vi "CODMn通讯.vi"() -> ()   [LabVIEW 2016, in "斯坦道CODMn.lvlib"]
uses:
  <vilib>/NI/Modbus Library/API/Wrapper/Create TCP Slave.vi
  <vilib>/NI/Modbus Library/API/slave/Modbus Slave.lvclass
  <vilib>/Plasmionique/MB Master/MB_Master/MB_Master.lvclass
  <vilib>/Plasmionique/MB Master/MB Master.lvlib
  <vilib>/Utility/config.llb/NI_LVConfig.lvlib
  <vilib>/NI/Modbus Library/API/Wrapper/API Main.lvlib
panel:
  in  "读取数据":bool
  in  "释放串口":bool
  in  "打开串口":bool
  out "队列中元素数量":i32
  out "元素":cluster{"命令":string}[](array[cluster])
  out "待处理插入数量":i32
  out "读取公式":u16[](array[numeric])
  out "读取参数":u16[](array[numeric])
  out "数据存储":u16[](array[numeric])
  out "温度":bool[](array[boolean])
  out "M输出点":bool[](array[boolean])
  out "ORP、时间":u16[](array[numeric])
  out "测量状态":u16[](array[numeric])
  out "通讯状态":bool
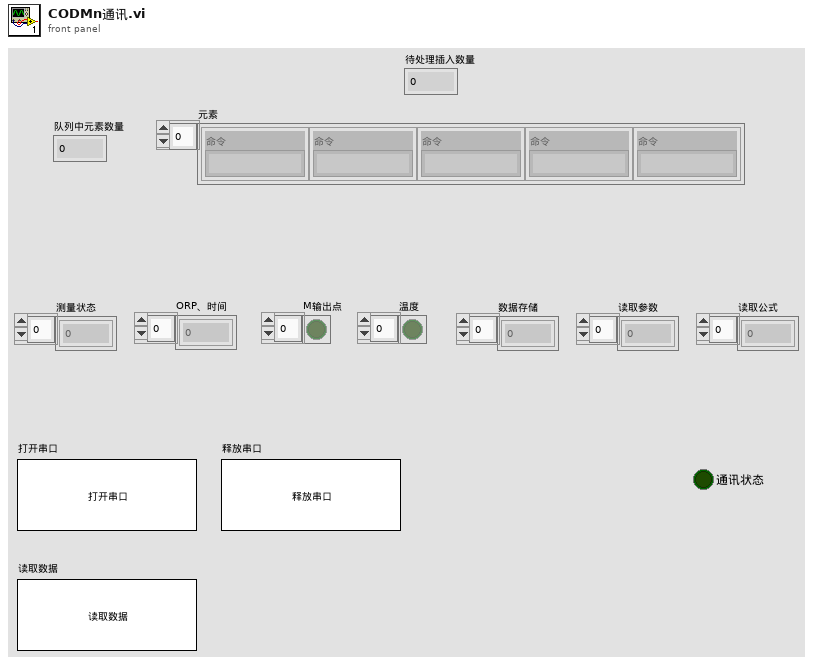
[diagram p1: front panel]
types:
  T1 = cluster{"命令":string, "测量模式":enum16{"水样测量", "标样核查", "零点核查", "跨度核查", "空白测试", "加标回收", "平行样", "校零", "校标"}, "CODMn量程切换":enum32{"H", "L", "AUTO"}}
  T2 = typedef "NI_LVConfig.lvlib/Config Data RefNum.ctl" = refnum<k1>
  T3 = enum16{"空闲", "水样测试", "标样核查", "零点核查", "跨度核查", "空白测试", "平行样测试", "质控样", "空白校准", "标样校准", "加标回收"}
  T4 = enum16{"水样测量", "标样核查", "零点核查", "跨度核查", "空白测试", "加标回收", "平行样", "校零", "校标"}
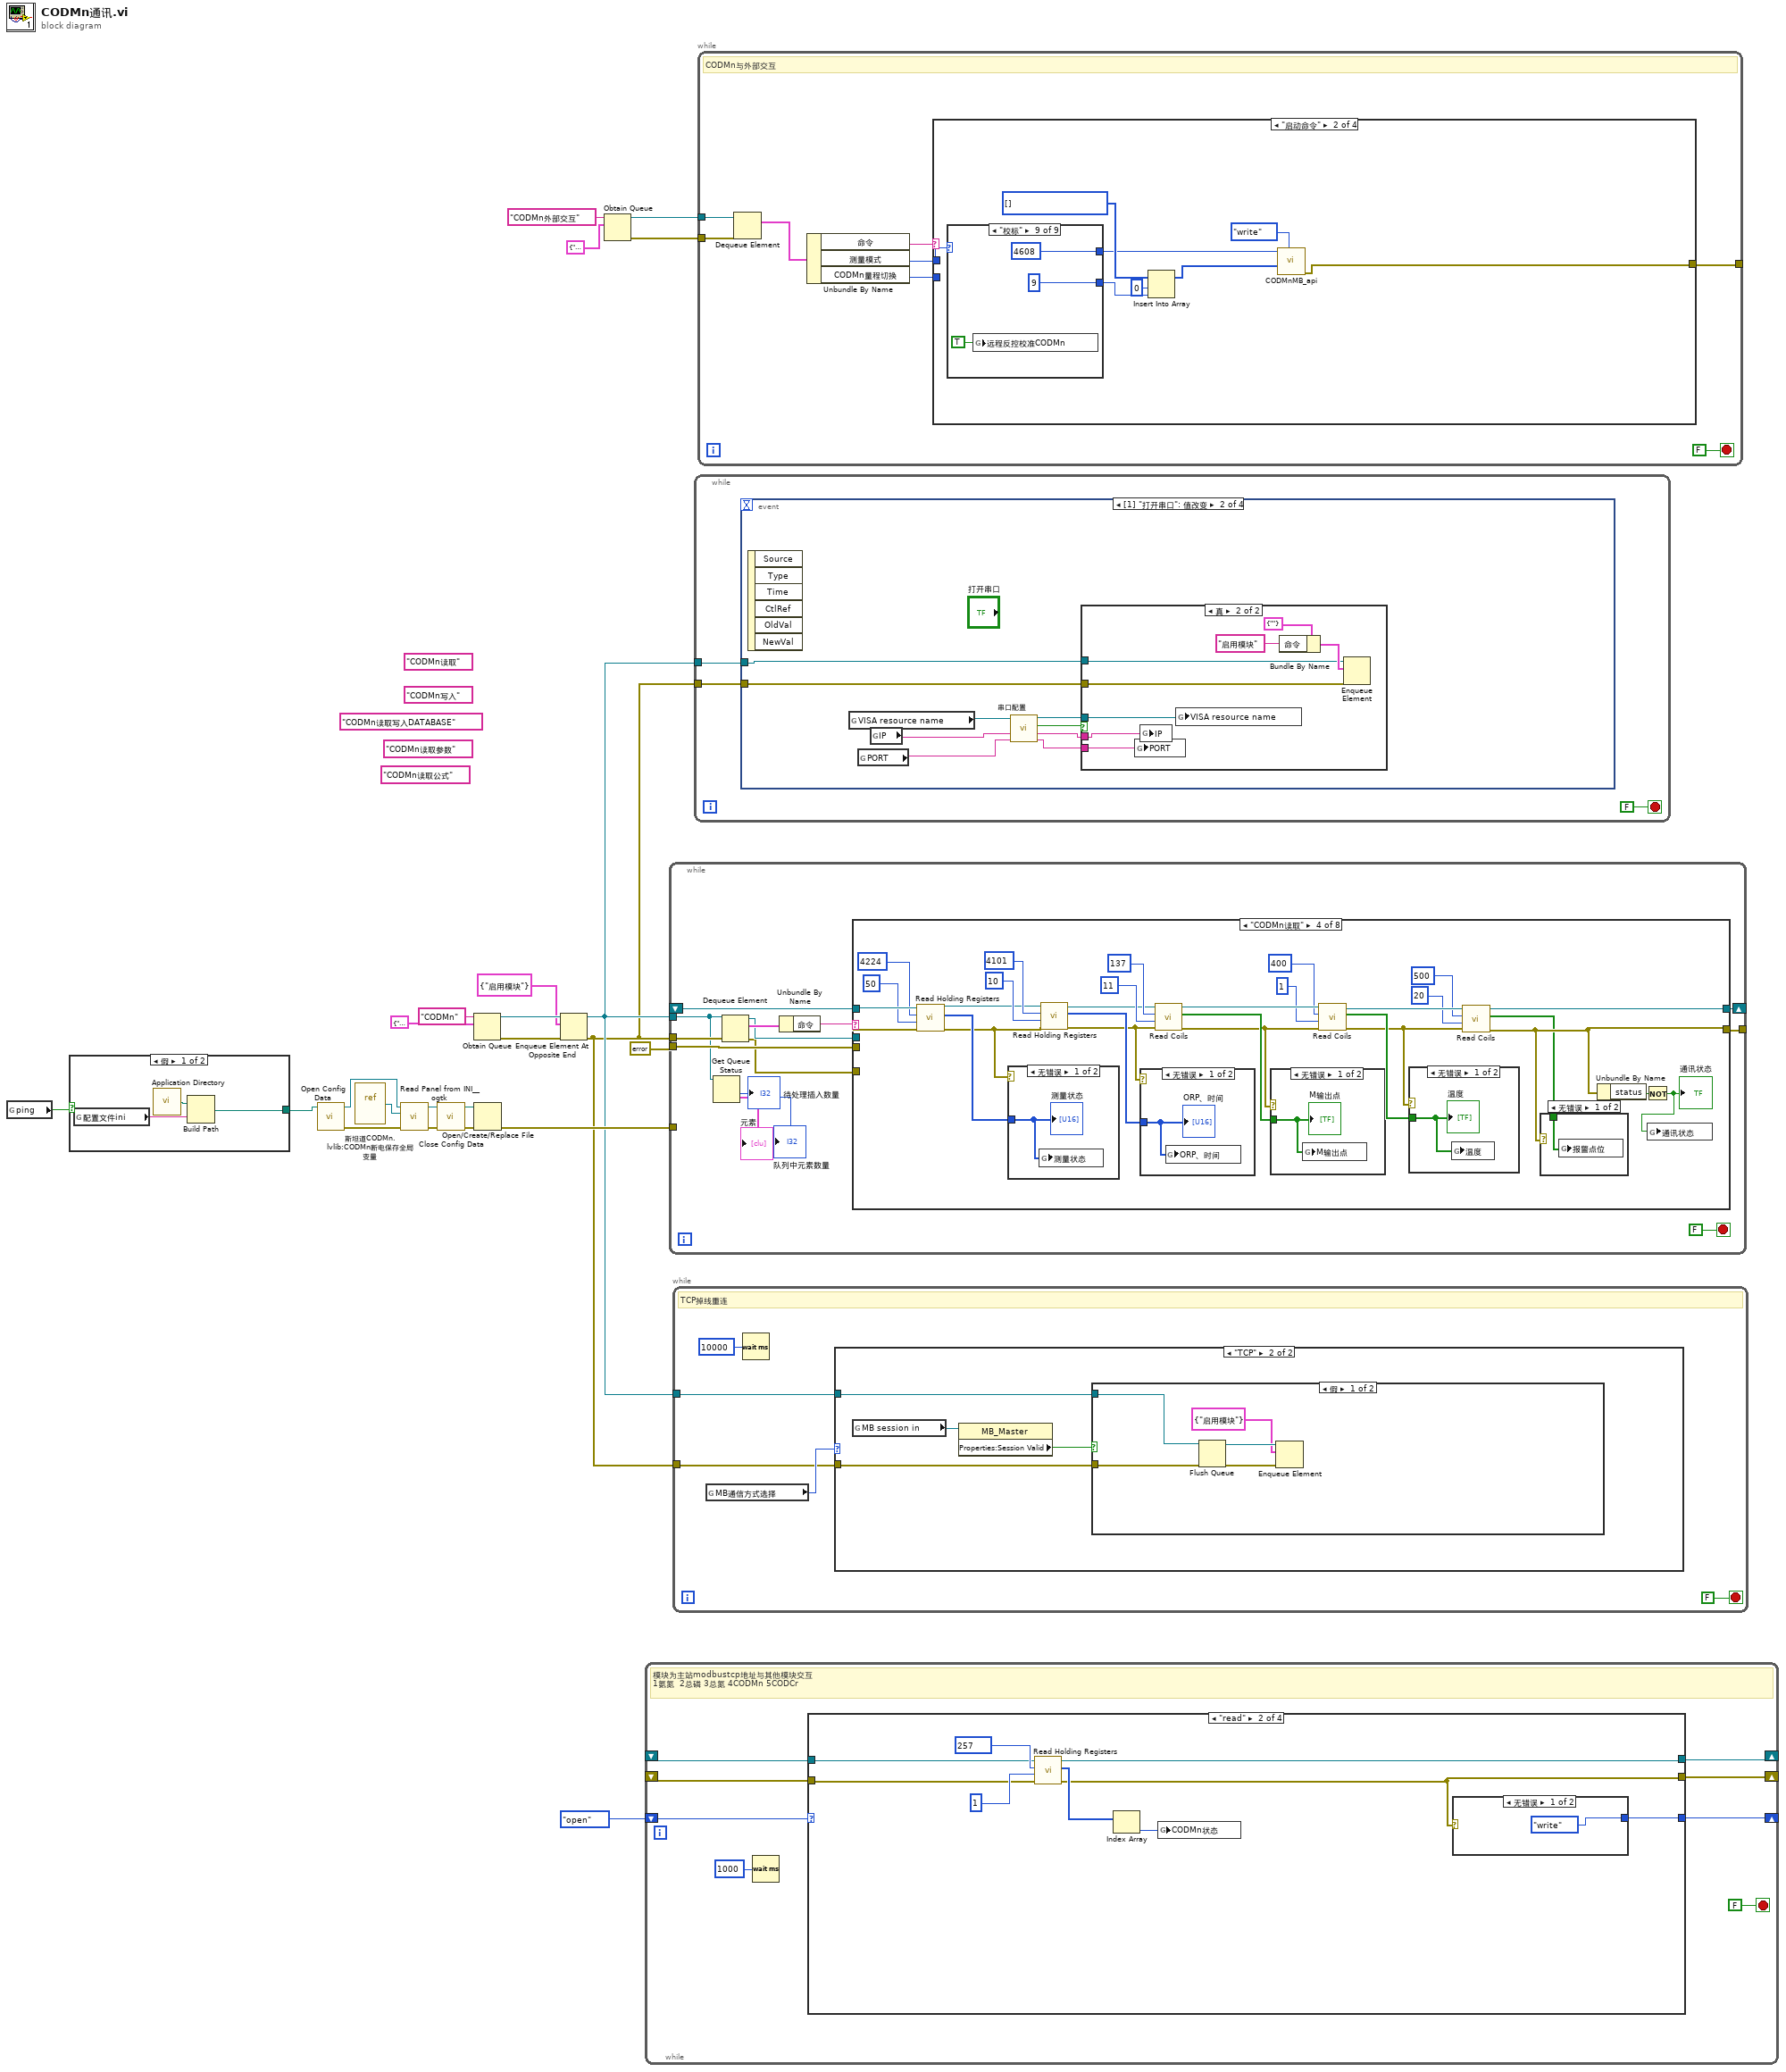
[diagram p0: block diagram]
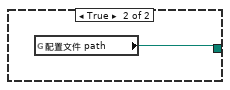
[diagram p2: hidden frame]
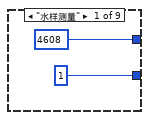
[diagram p4: hidden frame]
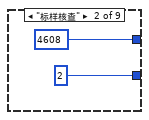
[diagram p5: hidden frame]
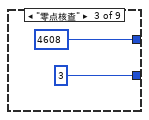
[diagram p6: hidden frame]
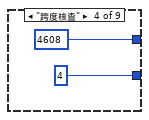
[diagram p7: hidden frame]
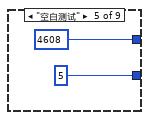
[diagram p8: hidden frame]
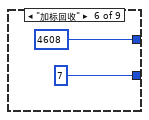
[diagram p9: hidden frame]
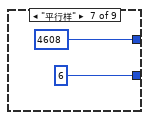
[diagram p10: hidden frame]
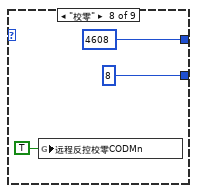
[diagram p11: hidden frame]
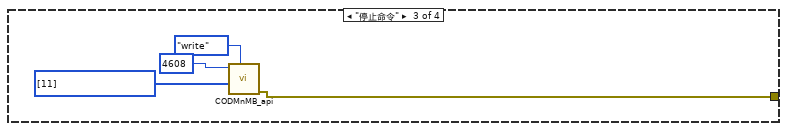
[diagram p12: hidden frame]
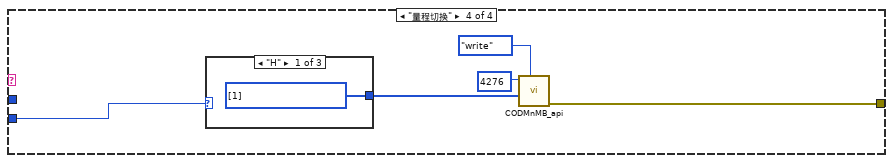
[diagram p13: hidden frame]
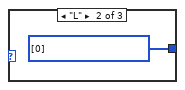
[diagram p14: hidden frame]
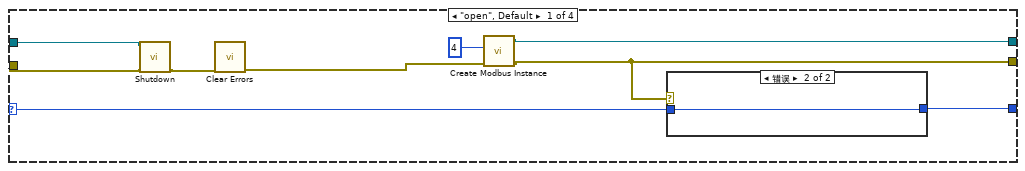
[diagram p18: hidden frame]
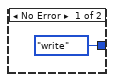
[diagram p19: hidden frame]
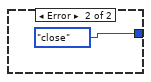
[diagram p20: hidden frame]
diagram:
  (unwired) "CODMn读取公式" ("名称（未命名）")
  (unwired) "CODMn读取写入DATABASE" ("名称（未命名）")
  (unwired) "CODMn读取参数" ("名称（未命名）")
  (unwired) "CODMn读取" ("名称（未命名）")
  (unwired) "CODMn写入" ("名称（未命名）")
  n1 = global read "CODMN外部API.vi" "ping"() -> (w2:bool)
  n2 = case shown="假" w2 {
    tunnel: [w24 w27] -> w1
    frame False {
      n3 = global read "COD内部交互全局.vi" "配置文件ini"() -> (w26:string)
      n4 = call <vilib>:"Application Directory.vi"() -> ("Application Directory"=w25:path)
      n5 = Build Path(base path=w25, name or relative path=w26) -> (appended path=w24:path)
    }
    frame True {
      n6 = global read "CODMN外部API.vi" "配置文件 path"() -> (w27:path)
    }
  }
  n7 = call <vilib>:"Open Config Data.vi"("configuration file path"=w1) -> ("error out"=w14:errorcluster, "refnum"=w17:T2)  [unwired: 8 in, 1 out]
  n8 = vi-ref "斯坦道CODMn.lvlib:CODMn断电保存全局变量.vi"() -> (w16:refnum<vi>)
  n9 = call <userlib>:"Read Panel from INI__ogtk.vi"("error in (no error)"=w14, "VI ref"=w16, "refnum"=w17) -> ("error out"=w13:errorcluster, "refnum out"=w15:T2)  [unwired: 7 in]
  n10 = call <vilib>:"Close Config Data.vi"("error in (no error)"=w13, "refnum"=w15) -> ("error out"=w12:errorcluster, "file path"=w11:path)  [unwired: 8 in]
  n11 = Obtain Queue(name (unnamed)="CODMn" ("名称（未命名）"), element data type=cluster{"命令":string} {"命令"="启用模块"} ("元素")) -> (queue out=w20:refnum<queue>, error out=w19:errorcluster)  [unwired: 3 in, 1 out]
  n12 = Open/Create/Replace File(file path (use dialog)=w11, error in=w12) -> (error out=w10:errorcluster)  [unwired: 4 in, 2 out]
  n13 = Enqueue Element At Opposite End(queue=w20, element=cluster{"命令":string} {"命令"="启用模块"} ("元素"), error in (no error)=w19) -> (queue out=w8:refnum<queue>, error out=w7:errorcluster)  [unwired: 1 in, 1 out]
  n14 = Obtain Queue(name (unnamed)="CODMn外部交互" ("名称（未命名）"), element data type=T1 {"命令"="启动命令", "测量模式"=enum."水样测量", "CODMn量程切换"=enum."AUTO"} ("元素")) -> (queue out=w4:refnum<queue>, error out=w3:errorcluster)  [unwired: 3 in, 1 out]
  n15 = while {
    shift-right: [w33] -> _
    shift-left: _ -> [w35]
    shift-right: [w32] -> _
    shift-left: _ -> [w34]
    shift-right: [w29] -> _
    shift-left: enum16{"open", "read", "write", "close"}."open" -> [w30]
    stop <- FALSE stop-if-true
    # "模块为主站modbustcp地址与其他模块交互\n1氨氮  2总磷 3总氮 4CODMn 5CODCr"
    n16 = Wait (ms)(milliseconds to wait=u32 1000 ("等待时间（毫秒）")) -> ()  [unwired: 1 out]
    n17 = case shown="\"read\"" w30 {
      selector: w30 -> [w44 _ _ _]
      tunnel: w35 -> [w38 w52 w75 w81]
      tunnel: w34 -> [w37 w51 w72 w80]
      tunnel: [w41 w47 w74 w81] -> w33
      tunnel: [w40 w48 w73 w83] -> w32
      tunnel: [w43 w55 w76 enum16{"open", "read", "write", "close"}."open"] -> w29
      frame "open", Default {
        n18 = call-dynamic "Shutdown.vi"("error in"=w37, "Modbus slave in"=w38) -> ("error out"=w36:errorcluster)  [unwired: 9 in]
        n19 = call <vilib>:"Clear Errors.vi"("error in (no error)"=w36) -> ("error out"=w39:errorcluster)  [unwired: 5 in, 1 out]
        n20 = call-poly <vilib>:"Create Modbus Instance.vi"("error in"=w39, "port (502)"=u16 4) -> ("error out"=w40:errorcluster, "TCP slave instance"=w41:refnum<class "Modbus Slave.lvclass">)  [unwired: 8 in]
        n21 = case shown="错误" w40 {
          tunnel: w44 -> [_ w46]
          tunnel: [enum16{"open", "read", "write", "close"}."write" w46] -> w43
          frame No Error {
          }
          frame Error {
          }
        }
      }
      frame "read" {
        n22 = call-dynamic <vilib>:"Read Holding Registers.vi"("error in"=w51, "number of inputs"=u16 1, "starting address"=u16 257, "Modbus slave in"=w52) -> ("error out"=w48:errorcluster, "register values"=w50:u16[], "Modbus slave out"=w47:refnum<class "Modbus Slave.lvclass">)  [unwired: 5 in]
        n23 = Index Array(array=w50) -> (element=w49:u16)  [unwired: 1 in]
        n24 = global write "CODMN外部API.vi" "CODMn状态"(w49) -> ()
        n25 = case shown="无错误" w48 {
          tunnel: [enum16{"open", "read", "write", "close"}."write" enum16{"open", "read", "write", "close"}."close"] -> w55
          frame No Error {
          }
          frame Error {
          }
        }
      }
      frame "write" {
        n26 = global read "COD测量模式全局.vi" "CODMn工作状态"() -> (w62:T3)
        n27 = global read "COD浓度全局变量.vi" "COD浓度（mg/L)"() -> (w64:dbl)
        n28 = global read "COD测量模式全局.vi" "加标回收启动时间"() -> (w67:timestamp)
        n29 = global read "COD测量模式全局.vi" "水样启动时间"() -> (w69:timestamp)
        n30 = global read "运行时序全局变量.vi" "多列列表框"() -> (w66:i32)
        n31 = Build Array(w69) -> (w68:timestamp[])
        n32 = Build Array(w64) -> (w63:dbl[])
        n33 = Build Array(w67) -> (w60:timestamp[])
        n34 = call "浮点转CDAB整形cod.vi"("浮点数"=w63) -> ("CDAB整形输出"=w65:u16[])  [unwired: 10 in]
        n35 = call "DateToHex.vi"("DATE"=w68) -> ("数组"=w71:u16[])  [unwired: 10 in]
        n36 = call "DateToHex.vi"("DATE"=w60) -> ("数组"=w70:u16[])  [unwired: 10 in]
        n37 = Insert Into Array(array=u16[] [] ("values"), new element #1=w62, new element #2=w65, new element #3=w66, new element #4=w70, new element #5=w71) -> (w59:u16[])  [unwired: 1 in]
        n38 = call-dynamic "Write Multiple Holding Registers.vi"("error in"=w72, "registers to write"=w59, "starting address"=u16 0, "Modbus slave in"=w75) -> ("error out"=w73:errorcluster, "Modbus slave out"=w74:refnum<class "Modbus Slave.lvclass">)  [unwired: 6 in]
        n39 = case shown="无错误" w73 {
          tunnel: [enum16{"open", "read", "write", "close"}."read" enum16{"open", "read", "write", "close"}."close"] -> w76
          frame No Error {
          }
          frame Error {
          }
        }
      }
      frame "close" {
        n40 = call-dynamic "Shutdown.vi"("error in"=w80, "Modbus slave in"=w81) -> ("error out"=w79:errorcluster)  [unwired: 9 in]
        n41 = call <vilib>:"Clear Errors.vi"("error in (no error)"=w79) -> ("error out"=w83:errorcluster)  [unwired: 5 in, 1 out]
      }
    }
  }
  n42 = while {
    tunnel: w8 -> [w89]
    tunnel: w7 -> [w96]
    tunnel: [w90] -> _
    shift-right: [w93] -> _
    shift-left: _ -> [w92]
    tunnel: errorcluster {"status"=FALSE, "code"=0, "source"=""} ("error out") -> [w91]
    tunnel: w10 -> [_]
    stop <- FALSE stop-if-true
    n43 = Get Queue Status(queue=w89) -> (# pending insert=→"待处理插入数量":i32, # elements in queue=→"队列中元素数量":i32, elements=→"元素":cluster{"命令":string}[])  [unwired: 2 in, 5 out]
    n44 = Dequeue Element(queue=w89, error in (no error)=w96) -> (queue out=w85:refnum<queue>, element=w95:cluster{"命令":string}, error out=w84:errorcluster)  [unwired: 1 in, 1 out]
    n45 = Unbundle By Name(w95) -> ("命令"=w94:string)
    n46 = case shown="\"CODMn读取\"" w94 {
      tunnel: [w99 w103 w114 w122 w154 w163 w180 w187] -> w93
      tunnel: [w98 w100 w115 w119 w152 w162 w179 w186] -> w90
      tunnel: w92 -> [w99 _ _ w146 w158 w172 w183 w191]
      tunnel: w91 -> [w98 w104 w116 w145 w155 w171 w182 w190]
      tunnel: w85 -> [_ w102 _ _ _ _ _ _]
      tunnel: w84 -> [_ w101 _ _ _ _ _ _]
      frame Default {
      }
      frame "启用模块" {
        n47 = call "CODMnMB_api.vi"("STEP"=enum16{"open", "read", "write", "close"}."open", "Error in"=w104) -> ("error out"=w100:errorcluster, "MB session out"=w103:refnum<class "MB_Master.lvclass">)  [unwired: 7 in, 1 out]
        n48 = case shown="无错误" w100 {
          tunnel: w102 -> [w110 _]
          tunnel: w101 -> [w107 _]
          frame No Error {
            n49 = global read "COD内部交互全局.vi" "序列号:"() -> (w109:string)
            n50 = Empty String/Path?(string/path=w109) -> (empty?=w108:bool)
            n51 = Not(x=w108) -> (.not. x?=w106:bool)
            n52 = case shown="真" w106 {
              tunnel: w110 -> [_ w113]
              tunnel: w107 -> [_ w112]
              frame False {
              }
              frame True {
                # "发货调试版用"
                n53 = Enqueue Element(queue=w113, element=cluster{"命令":string} {"命令"="CODMn序列号写入"} ("元素"), error in (no error)=w112) -> ()  [unwired: 1 in, 3 out]
              }
            }
          }
          frame Error {
          }
        }
        n54 = global write "COD浓度全局变量.vi" "MB session in"(w103) -> ()
      }
      frame "停用模块" {
        n55 = call "CODMnMB_api.vi"("STEP"=enum16{"open", "read", "write", "close"}."close", "Error in"=w116) -> ("error out"=w115:errorcluster, "MB session out"=w114:refnum<class "MB_Master.lvclass">)  [unwired: 7 in, 1 out]
      }
      frame "CODMn读取" {
        n56 = call <vilib>:"Read Holding Registers.vi"("error in (no error)"=w145, "quantity"=u16 50 ("number of holding registers"), "starting address"=u16 4224, "MB session in"=w146) -> ("error out"=w136:errorcluster, "Registers"=w142:u16[], "MB session out"=w137:refnum<class "MB_Master.lvclass">)  [unwired: 5 in]
        n57 = case shown="无错误" w136 {
          tunnel: w142 -> [w151 _]
          frame No Error {
            n58 = global write "COD内部交互全局.vi" "测量状态"(w151) -> ()
            "测量状态" <- w151
          }
          frame Error {
          }
        }
        n59 = call <vilib>:"Read Holding Registers.vi"("error in (no error)"=w136, "quantity"=u16 10, "starting address"=u16 4101, "MB session in"=w137) -> ("error out"=w132:errorcluster, "Registers"=w135:u16[], "MB session out"=w134:refnum<class "MB_Master.lvclass">)  [unwired: 5 in]
        n60 = case shown="无错误" w132 {
          tunnel: w135 -> [w150 _]
          frame No Error {
            n61 = global write "COD内部交互全局.vi" "ORP、时间"(w150) -> ()
            "ORP、时间" <- w150
          }
          frame Error {
          }
        }
        n62 = call <vilib>:"Read Coils.vi"("error in (no error)"=w132, "quantity"=u16 11, "starting address"=u16 137, "MB session in"=w134) -> ("error out"=w130:errorcluster, "Coils"=w131:bool[], "MB session out"=w133:refnum<class "MB_Master.lvclass">)  [unwired: 5 in]
        n63 = case shown="无错误" w130 {
          tunnel: w131 -> [w149 _]
          frame No Error {
            n64 = global write "COD内部交互全局.vi" "M输出点"(w149) -> ()
            "M输出点" <- w149
          }
          frame Error {
          }
        }
        n65 = call <vilib>:"Read Coils.vi"("error in (no error)"=w130, "quantity"=u16 1, "starting address"=u16 400, "MB session in"=w133) -> ("error out"=w123:errorcluster, "Coils"=w127:bool[], "MB session out"=w124:refnum<class "MB_Master.lvclass">)  [unwired: 5 in]
        n66 = case shown="无错误" w123 {
          tunnel: w127 -> [w148 _]
          frame No Error {
            n67 = global write "COD内部交互全局.vi" "温度"(w148) -> ()
            "温度" <- w148
          }
          frame Error {
          }
        }
        n68 = call <vilib>:"Read Coils.vi"("error in (no error)"=w123, "quantity"=u16 20, "starting address"=u16 500, "MB session in"=w124) -> ("error out"=w119:errorcluster, "Coils"=w118:bool[], "MB session out"=w122:refnum<class "MB_Master.lvclass">)  [unwired: 5 in]
        n69 = case shown="无错误" w119 {
          tunnel: w118 -> [w147 _]
          frame No Error {
            n70 = global write "COD内部交互全局.vi" "报警点位"(w147) -> ()
          }
          frame Error {
          }
        }
        n71 = Unbundle By Name(w119) -> ("status"=w126:bool)
        n72 = Not(x=w126) -> (.not. x?=w125:bool)
        "通讯状态" <- w125
        n73 = global write "COD内部交互全局.vi" "通讯状态"(w125) -> ()
      }
      frame "CODMn读取写入DATABASE" {
        n74 = call <vilib>:"Read Holding Registers.vi"("error in (no error)"=w155, "quantity"=u16 10 ("number of holding registers"), "starting address"=u16 4101, "MB session in"=w158) -> ("error out"=w152:errorcluster, "Registers"=w153:u16[], "MB session out"=w154:refnum<class "MB_Master.lvclass">)  [unwired: 5 in]
        n75 = case shown="无错误" w152 {
          tunnel: w153 -> [w160 _]
          frame No Error {
            n76 = global write "COD内部交互全局.vi" "数据存储"(w160) -> ()
            n77 = global write "COD内部交互全局.vi" "读取写入data"(TRUE ("读取参数显示")) -> ()
            "数据存储" <- w160
          }
          frame Error {
          }
        }
      }
      frame "CODMn读取参数" {
        n78 = call <vilib>:"Read Holding Registers.vi"("error in (no error)"=w171, "quantity"=u16 35 ("number of holding registers"), "starting address"=u16 4272, "MB session in"=w172) -> ("error out"=w166:errorcluster, "Registers"=w168:u16[], "MB session out"=w167:refnum<class "MB_Master.lvclass">)  [unwired: 5 in]
        n79 = case shown="无错误" w166 {
          tunnel: w168 -> [w176 _]
          frame No Error {
            n80 = global write "COD内部交互全局.vi" "读取参数"(w176) -> ()
            n81 = global write "COD内部交互全局.vi" "读取参数显示"(TRUE ("读取参数显示")) -> ()
            "读取参数" <- w176
          }
          frame Error {
          }
        }
        n82 = call <vilib>:"Read Holding Registers.vi"("error in (no error)"=w166, "quantity"=u16 4, "starting address"=u16 5596, "MB session in"=w167) -> ("error out"=w162:errorcluster, "Registers"=w161:u16[], "MB session out"=w163:refnum<class "MB_Master.lvclass">)  [unwired: 5 in]
        n83 = case shown="无错误" w162 {
          tunnel: w161 -> [w174 _]
          frame No Error {
            n84 = global write "COD内部交互全局.vi" "读取浮台参数"(w174) -> ()
            n85 = global write "COD内部交互全局.vi" "读取浮台参数显示"(TRUE ("读取参数显示")) -> ()
          }
          frame Error {
          }
        }
      }
      frame "CODMn读取公式" {
        n86 = call <vilib>:"Read Holding Registers.vi"("error in (no error)"=w182, "quantity"=u16 94 ("number of holding registers"), "starting address"=u16 4616, "MB session in"=w183) -> ("error out"=w179:errorcluster, "Registers"=w181:u16[], "MB session out"=w180:refnum<class "MB_Master.lvclass">)  [unwired: 5 in]
        n87 = case shown="无错误" w179 {
          tunnel: w181 -> [w185 _]
          frame No Error {
            n88 = global write "COD内部交互全局.vi" "读取公式"(w185) -> ()
            n89 = global write "COD内部交互全局.vi" "读取公式显示"(TRUE ("读取参数显示")) -> ()
            "读取公式" <- w185
          }
          frame Error {
          }
        }
      }
      frame "CODMn序列号写入" {
        n90 = global read "COD内部交互全局.vi" "序列号:"() -> (w189:string)
        n91 = call "StringToHex.vi"("STRING"=w189) -> ("数组"=w188:u16[])  [unwired: 10 in]
        n92 = call <vilib>:"Write Multiple Registers.vi"("error in (no error)"=w190, "values"=w188, "starting address"=u16 4298, "MB session in"=w191) -> ("error out"=w186:errorcluster, "MB session out"=w187:refnum<class "MB_Master.lvclass">)  [unwired: 6 in]
      }
    }
  }
  n93 = while "While循环" {
    tunnel: w8 -> [w194]
    tunnel: w7 -> [w193]
    stop <- FALSE stop-if-true
    # "TCP掉线重连"
    n94 = global read "CODMn断电保存全局变量.vi" "MB通信方式选择"() -> (w195:enum16{"串口", "TCP"})
    n95 = Wait (ms)(milliseconds to wait=u32 10000 ("等待时间（毫秒）")) -> ()  [unwired: 1 out]
    n96 = case shown="\"TCP\"" w195 {
      tunnel: w194 -> [_ w199]
      tunnel: w193 -> [_ w198]
      frame "串口", Default {
      }
      frame "TCP" {
        n97 = global read "COD浓度全局变量.vi" "MB session in"() -> (w201:refnum<class "MB_Master.lvclass">)
        n98 = property class="MB_Master"(reference=w201) -> ("Properties:Session Valid"=w200:bool)  [unwired: 1 in, 2 out]
        n99 = case shown="假" w200 {
          tunnel: w199 -> [w203 _]
          tunnel: w198 -> [w202 _]
          frame False {
            n100 = Flush Queue(queue=w203, error in (no error)=w202) -> (queue out=w206:refnum<queue>, error out=w205:errorcluster)  [unwired: 1 out]
            n101 = Enqueue Element(queue=w206, element=cluster{"命令":string} {"命令"="启用模块"} ("元素"), error in (no error)=w205) -> ()  [unwired: 1 in, 3 out]
          }
          frame True {
          }
        }
      }
    }
  }
  n102 = while {
    tunnel: w8 -> [w208]
    tunnel: w7 -> [w207]
    stop <- FALSE stop-if-true
    n103 = event shown="[1] \"打开串口\": 值改变" {
      selector: _ -> [_ _ _ _]
      dyn-events: _ -> [_ _ _ _]
      timeout: _ -> [_ _ _ _]
      tunnel: w208 -> [_ w215 w229 w231]
      tunnel: w207 -> [_ w214 w228 w230]
      event Timeout {
        n104 = event-data() -> ()  [unwired: 1 in, 3 out]
      }
      event "打开串口": Value Change {
        n105 = event-data() -> ()  [unwired: 1 in, 6 out]
        n106 = global read "CODMn断电保存全局变量.vi" "VISA resource name"() -> (w218:refnum<visa-resource-name>)
        n107 = global read "CODMn断电保存全局变量.vi" "PORT"() -> (w210:string)
        n108 = global read "CODMn断电保存全局变量.vi" "IP"() -> (w211:string)
        n109 = call "串口配置.vi"("PORT"=w210, "IP"=w211, "请选择串口:"=w218) -> ("PORT 2"=w212:string, "IP 2"=w213:string, "确认 2"=w216:bool, "VISA资源名称 2"=w217:refnum<visa-resource-name>)  [unwired: 4 in, 1 out]
        n110 = case shown="真" w216 {
          tunnel: w217 -> [_ w226]
          tunnel: w215 -> [_ w222]
          tunnel: w214 -> [_ w221]
          tunnel: w213 -> [_ w220]
          tunnel: w212 -> [_ w219]
          frame False {
          }
          frame True {
            n111 = global write "CODMn断电保存全局变量.vi" "PORT"(w219) -> ()
            n112 = global write "CODMn断电保存全局变量.vi" "IP"(w220) -> ()
            n113 = global write "CODMn断电保存全局变量.vi" "VISA resource name"(w226) -> ()
            n114 = Bundle By Name(cluster=cluster{"命令":string} {"命令"=""} ("元素"), "命令"="启用模块" ("名称（未命名）")) -> (w223:cluster{"命令":string})
            n115 = Enqueue Element(queue=w222, element=w223, error in (no error)=w221) -> ()  [unwired: 1 in, 3 out]
          }
        }
      }
      event "释放串口": Value Change {
        n116 = event-data() -> ()  [unwired: 1 in, 6 out]
        n117 = Enqueue Element(queue=w229, element=cluster{"命令":string} {"命令"="停用模块"} ("元素"), error in (no error)=w228) -> ()  [unwired: 1 in, 3 out]
      }
      event "读取数据": Value Change {
        n118 = event-data() -> ()  [unwired: 1 in, 6 out]
        n119 = Enqueue Element(queue=w231, element=cluster{"命令":string} {"命令"="CODMn读取"} ("元素"), error in (no error)=w230) -> ()  [unwired: 1 in, 3 out]
      }
    }
  }
  n120 = while {
    tunnel: w4 -> [w238]
    tunnel: w3 -> [w237]
    tunnel: [w233] -> _
    stop <- FALSE stop-if-true
    # "CODMn与外部交互"
    n121 = Dequeue Element(queue=w238, error in (no error)=w237) -> (element=w239:T1)  [unwired: 1 in, 3 out]
    n122 = Unbundle By Name(w239) -> ("命令"=w236:string, "测量模式"=w235:T4, "CODMn量程切换"=w234:enum32{"H", "L", "AUTO"})
    n123 = case shown="\"启动命令\"" w236 {
      tunnel: w235 -> [_ w242 _ _]
      tunnel: w234 -> [_ _ _ w274]
      tunnel: [_ w241 w269 w273] -> w233
      frame "假", Default {
      }
      frame "启动命令" {
        n124 = case shown="\"校标\"" w242 {
          tunnel: [u16 4608 ("address") u16 4608 ("address") u16 4608 ("address") u16 4608 ("address") u16 4608 ("address") u16 4608 ("address") u16 4608 ("address") u16 4608 ("address") u16 4608 ("address")] -> w244
          tunnel: [u16 1 ("address") u16 2 ("address") u16 3 ("address") u16 4 ("address") u16 5 ("address") u16 7 ("address") u16 6 ("address") u16 8 ("address") u16 9 ("address")] -> w248
          frame "水样测量" {
          }
          frame "标样核查" {
          }
          frame "零点核查" {
          }
          frame "跨度核查" {
          }
          frame "空白测试" {
          }
          frame "加标回收" {
          }
          frame "平行样" {
          }
          frame "校零" {
            n125 = global write "CODMN外部API.vi" "远程反控校零CODMn"(TRUE ("远程反控校准CODMn")) -> ()
          }
          frame "校标" {
            n126 = global write "CODMN外部API.vi" "远程反控校准CODMn"(TRUE ("远程反控校准CODMn")) -> ()
          }
        }
        n127 = Insert Into Array(array=u16[] [] ("values"), index=0 ("索引"), new element=w248) -> (w243:u16[])
        n128 = call "CODMnMB_api.vi"("STEP"=enum16{"open", "read", "write", "close"}."write", "values"=w243, "starting address"=w244) -> ("error out"=w241:errorcluster)  [unwired: 6 in, 2 out]
      }
      frame "停止命令" {
        n129 = call "CODMnMB_api.vi"("STEP"=enum16{"open", "read", "write", "close"}."write", "values"=u16[] [11], "starting address"=u16 4608) -> ("error out"=w269:errorcluster)  [unwired: 6 in, 2 out]
      }
      frame "量程切换" {
        n130 = case shown="\"H\"" w274 {
          tunnel: [u16[] [1] ("values") u16[] [0] ("values") _] -> w277
          frame "H" {
          }
          frame "L" {
          }
          frame "AUTO", Default {
          }
        }
        n131 = call "CODMnMB_api.vi"("STEP"=enum16{"open", "read", "write", "close"}."write", "values"=w277, "starting address"=u16 4276) -> ("error out"=w273:errorcluster)  [unwired: 6 in, 2 out]
      }
    }
  }
